vi "Move_LDA_Mirror.vi"(4 "Mirror Up?":bool=TRUE) -> (0 "Error Message":string)   [LabVIEW 2020]
uses:
  Controls/User_Specific_mode.ctl
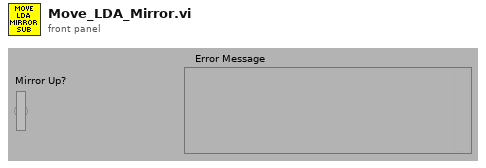
[diagram p1: front panel]
types:
  T1 = typedef "User_Specific_mode.ctl" = enum16{"Check VI only", "Run VI"}
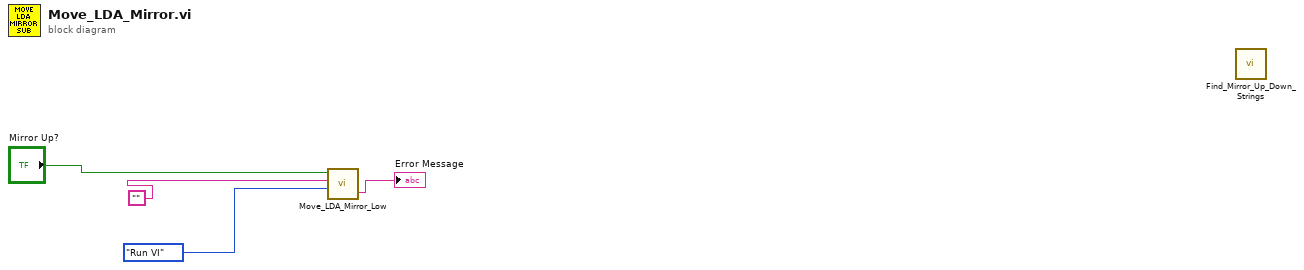
[diagram p0: block diagram]
diagram:
  n1 = call "Move_LDA_Mirror_Low.vi"("Mode"=User_Specific_mode."Run VI", "Extra Commands"="", "Mirror Up?"="Mirror Up?") -> ("Error Message"=→"Error Message":string)  [unwired: 1 in, 1 out]
  n2 = call "Find_Mirror_Up_Down_Strings.vi"() -> ()  [unwired: 2 in, 2 out]
